vi "Reqs2Bool.vi"(8 "error_in":errorcluster, 11 "Requirements":T1) -> (0 "error_out":errorcluster, 2 "Requeriments_boolean":T2)   [LabVIEW 2017]
uses:
  CONTROLS/Requirements_boolean.ctl
  CONTROLS/Requirements.ctl
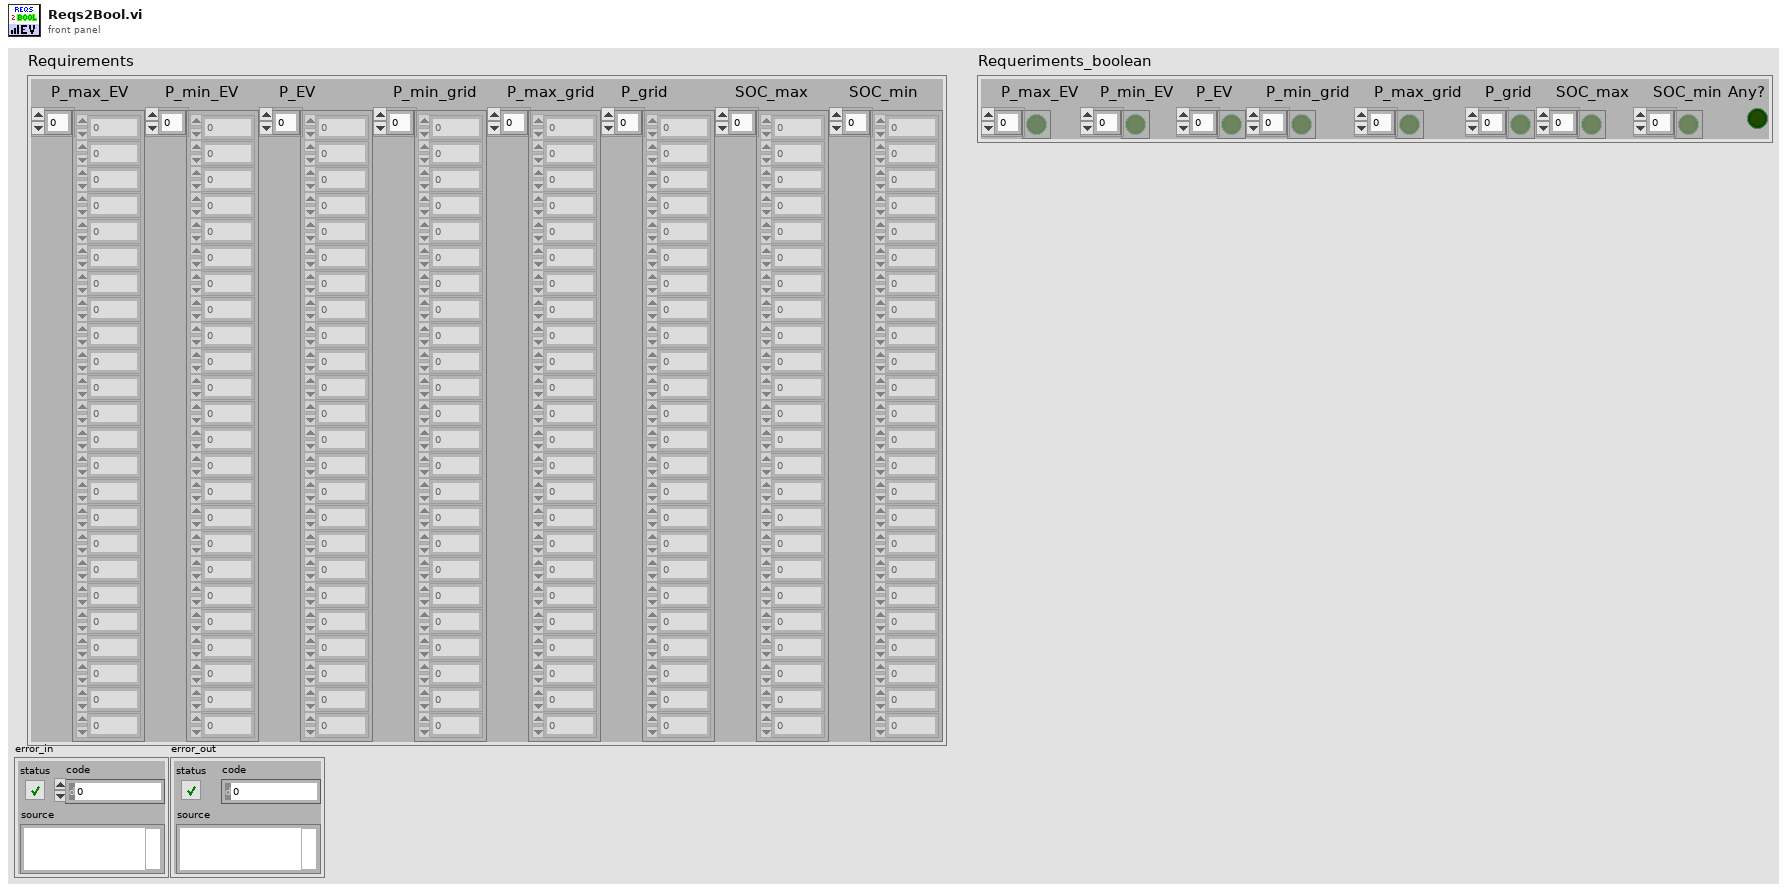
[diagram p1: front panel]
types:
  T1 = typedef "Requirements.ctl" = cluster{"P_max_EV":dbl[], "P_min_EV":dbl[], "P_EV":dbl[], "P_min_grid":dbl[], "P_max_grid":dbl[], "P_grid":dbl[], "SOC_max":dbl[], "SOC_min":dbl[]}
  T2 = typedef "Requirements_boolean.ctl" = cluster{"P_max_EV":bool[], "P_min_EV":bool[], "P_EV":bool[], "P_min_grid":bool[], "P_max_grid":bool[], "P_grid":bool[], "SOC_max":bool[], "SOC_min":bool[], "Any?":bool}
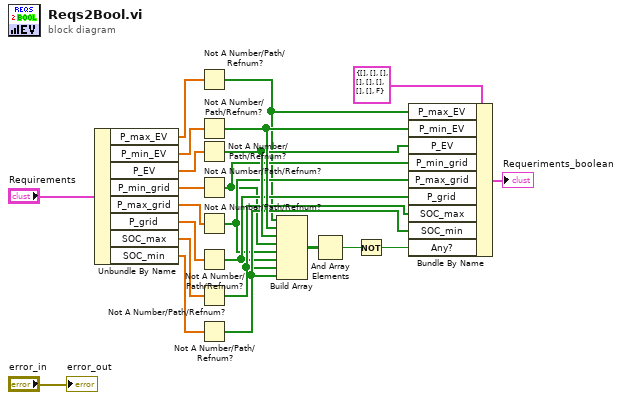
[diagram p0: block diagram]
diagram:
  n1 = Unbundle By Name("Requirements") -> ("P_max_EV"=w3:dbl[], "P_min_EV"=w4:dbl[], "P_EV"=w5:dbl[], "P_min_grid"=w8:dbl[], "P_max_grid"=w7:dbl[], "P_grid"=w9:dbl[], "SOC_max"=w11:dbl[], "SOC_min"=w10:dbl[])
  n2 = Not A Number/Path/Refnum?(number/path/refnum=w3) -> (NaN/Path/Refnum?=w14:bool[])
  n3 = Not A Number/Path/Refnum?(number/path/refnum=w4) -> (NaN/Path/Refnum?=w21:bool[])
  n4 = Not A Number/Path/Refnum?(number/path/refnum=w5) -> (NaN/Path/Refnum?=w20:bool[])
  n5 = Not A Number/Path/Refnum?(number/path/refnum=w8) -> (NaN/Path/Refnum?=w15:bool[])
  n6 = Not A Number/Path/Refnum?(number/path/refnum=w7) -> (NaN/Path/Refnum?=w16:bool[])
  n7 = Not A Number/Path/Refnum?(number/path/refnum=w9) -> (NaN/Path/Refnum?=w17:bool[])
  n8 = Not A Number/Path/Refnum?(number/path/refnum=w11) -> (NaN/Path/Refnum?=w18:bool[])
  n9 = Not A Number/Path/Refnum?(number/path/refnum=w10) -> (NaN/Path/Refnum?=w19:bool[])
  n10 = Build Array(w14, w21, w20, w15, w16, w17, w18, w19) -> (w2:bool[][])
  n11 = And Array Elements(Boolean array=w2) -> (logical AND=w6:bool)
  n12 = Not(x=w6) -> (.not. x?=w23:bool)
  n13 = Bundle By Name(cluster=T2 {"P_max_EV"=[], "P_min_EV"=[], "P_EV"=[], "P_min_grid"=[], "P_max_grid"=[], "P_grid"=[], "SOC_max"=[], "SOC_min"=[], "Any?"=FALSE} ("Requeriments_boolean"), "P_max_EV"=w14, "P_min_EV"=w21, "P_EV"=w20, "P_min_grid"=w15, "P_max_grid"=w16, "P_grid"=w17, "SOC_max"=w18, "SOC_min"=w19, "Any?"=w23) -> (→"Requeriments_boolean":T2)
  "error_out" <- "error_in"
